vi "ClientKey.vi"(9 "HMAC parameters":T1, 10 "Un-hashed client Key":string, 11 "Secret":string) -> (3 "ClientKey":u8[](array[numeric]))   [LabVIEW 2020, in "wamplv.lvlib" / "WampScramAuthenticator.lvclass"]
uses:
  WampScramAuthenticator.lvclass
  WampScramAuthenticator.lvclass/WampScramAuthenticator.ctl
  HashLib/HashLib.lvclass
  Utils/Utils.lvclass
  TypeDefs/HMAC parameters.ctl
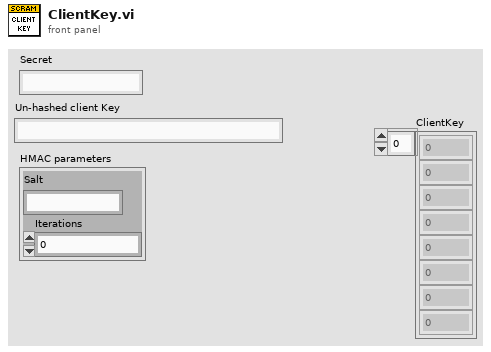
[diagram p1: front panel]
types:
  T1 = typedef "wamplv.lvlib/WampScramAuthenticator.lvclass/HMAC parameters.ctl" = cluster{"Salt":string, "Iterations":i32}
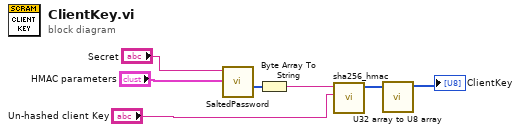
[diagram p0: block diagram]
diagram:
  n1 = call "SaltedPassword.vi"("HMAC parameters"="HMAC parameters", "Secret"="Secret") -> ("Salted password"=w3:u8[])  [unwired: 9 in]
  n2 = Byte Array To String(unsigned byte array=w3) -> (string=w2:string)
  n3 = call "sha256_hmac.vi"("data"="Un-hashed client Key", "key"=w2) -> ("sha256"=w1:u32[])  [unwired: 9 in]
  n4 = call "U32 array to U8 array.vi"("Array in"=w1) -> ("Array out"=→"ClientKey":u8[])  [unwired: 10 in]
